vi "MapLocalToRemotePath.vi"(10 "appref":refnum<vi>, 11 "local path":path) -> (3 "remote path":path)   [LabVIEW 2020, in "NI_TargetHelper.lvlib" / "NetCPU.lvclass"]
uses:
  <vilib>/TargetSupport/NI_TargetHelper/NetCPU/NetCPU.lvclass
  <vilib>/Utility/sysdir.llb/System Directory Type.ctl
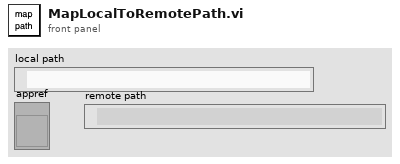
[diagram p1: front panel]
types:
  T1 = typedef "System Directory Type.ctl" = i32
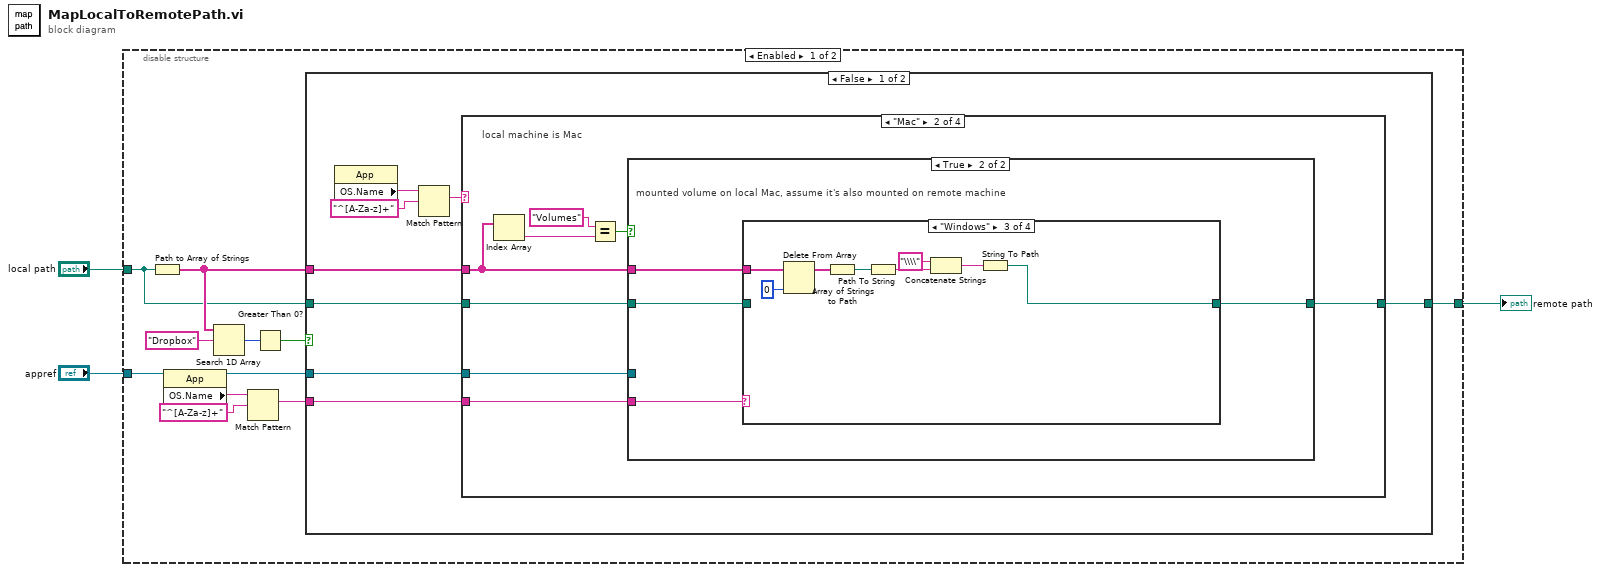
[diagram p0: block diagram]
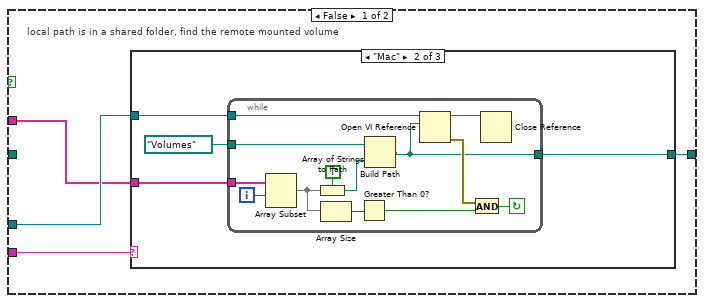
[diagram p3: hidden frame]
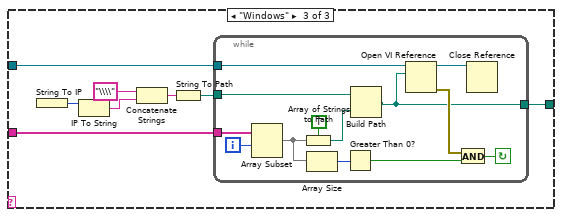
[diagram p5: hidden frame]
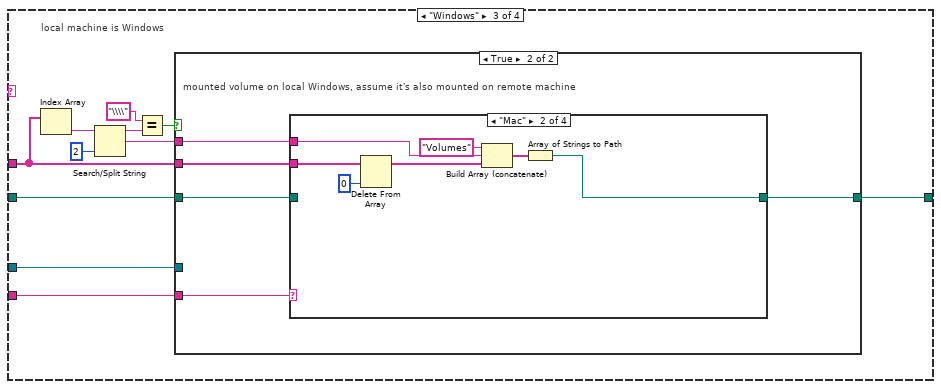
[diagram p9: hidden frame]
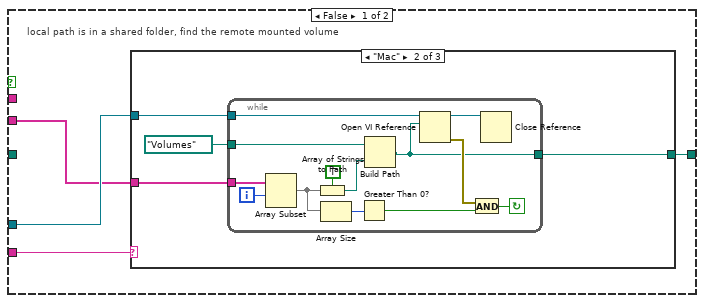
[diagram p10: hidden frame]
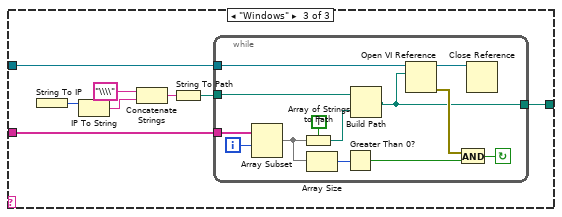
[diagram p12: hidden frame]
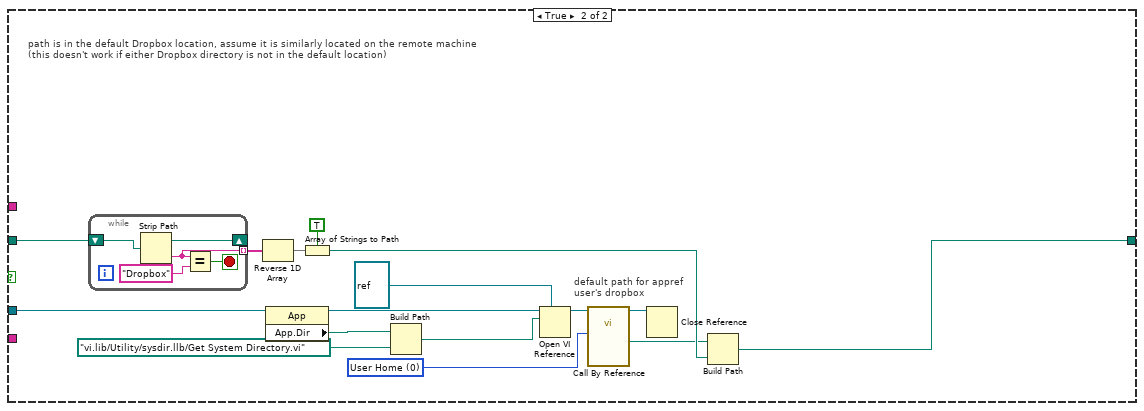
[diagram p17: hidden frame]
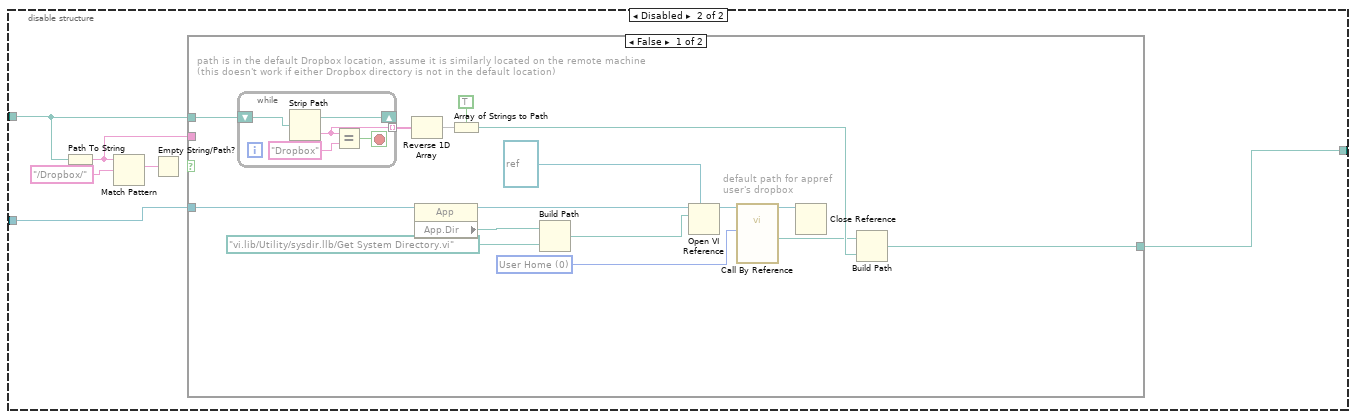
[diagram p18: hidden frame]
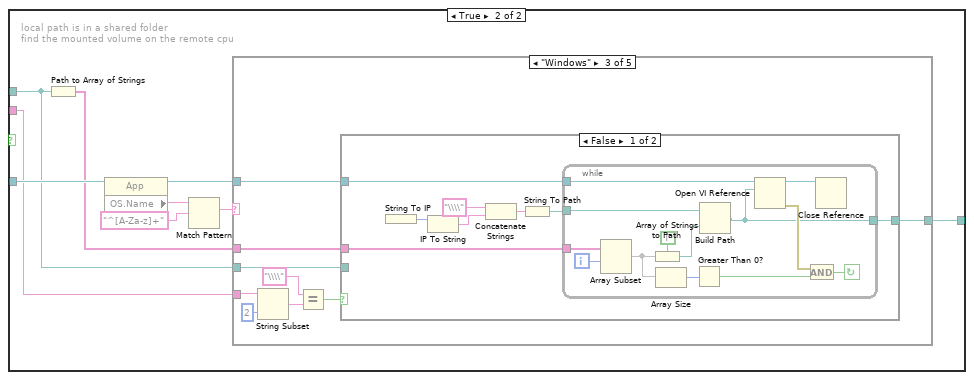
[diagram p19: hidden frame]
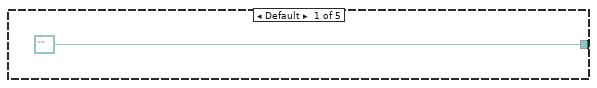
[diagram p20: hidden frame]
diagram:
  n1 = disable-structure shown="Enabled" {
    disable-tunnel: "appref" -> [w12 w174]
    disable-tunnel: "local path" -> [w4 w175]
    disable-tunnel: [w5 w173] -> w1
    frame Enabled {
      n2 = Path to Array of Strings(0:w4) -> (2:w7:string[])  [unwired: 1 out]
      n3 = property class="App"(reference=w12) -> (reference out=w10:refnum<vi>, "OS.Name"=w13:string)  [unwired: 1 in, 1 out]
      n4 = Search 1D Array(1D array=w7, element="Dropbox") -> (index of element=w9:i32)  [unwired: 1 in]
      n5 = Match Pattern(string=w13, regular expression="^[A-Za-z]+") -> (match substring=w11:string)  [unwired: 1 in, 3 out]
      n6 = Greater Than 0?(x=w9) -> (x > 0?=w6:bool)
      n7 = case shown="False" w6 {
        tunnel: w11 -> [w15 _]
        tunnel: w10 -> [w19 w153]
        tunnel: w4 -> [w18 w154]
        tunnel: w7 -> [w17 _]
        tunnel: [w16 w152] -> w5
        frame False {
          n8 = property class="App"() -> ("OS.Name"=w22:string)  [unwired: 2 in, 2 out]
          n9 = Match Pattern(string=w22, regular expression="^[A-Za-z]+") -> (match substring=w20:string)  [unwired: 1 in, 3 out]
          n10 = case shown="\"Mac\"" w20 {
            tunnel: w18 -> [_ w25 w92 _]
            tunnel: w15 -> [_ w27 w94 _]
            tunnel: [_ w26 w93 _] -> w16
            tunnel: w19 -> [_ w24 w91 _]
            tunnel: w17 -> [_ w23 w86 _]
            frame Default {
            }
            frame "Mac" {
              # "local machine is Mac"
              n11 = Index Array(array=w23) -> (element=w30:string)  [unwired: 1 in]
              n12 = Equal?(x="Volumes" ("y"), y=w30) -> (x = y?=w28:bool)
              n13 = case shown="True" w28 {
                tunnel: w27 -> [w32 w76]
                tunnel: [w31 w75] -> w26
                tunnel: w25 -> [_ w74]
                tunnel: w23 -> [w33 w73]
                tunnel: w24 -> [w34 _]
                frame False {
                  # "local path is in a shared folder, find the remote mounted volume"
                  n14 = case shown="\"Mac\"" w32 {
                    tunnel: w34 -> [_ w37 w53]
                    tunnel: w33 -> [_ w36 w52]
                    tunnel: [_ w35 w54] -> w31
                    frame Default {
                    }
                    frame "Mac" {
                      n15 = while {
                        tunnel: path "/Volumes" -> [w51]
                        tunnel: w37 -> [w50]
                        tunnel: w36 -> [w49]
                        tunnel: [w40] -> w35
                        i -> [w48]
                        stop <- w42 continue-if-true
                        n16 = Array Subset(array=w49, index=w48) -> (w46:string[])  [unwired: 1 in]
                        n17 = Array of Strings to Path(0:w46, 1:TRUE ("relative")) -> (2:w47:path)
                        n18 = Array Size(array=w46) -> (size(s)=w45:i32)
                        n19 = Greater Than 0?(x=w45) -> (x > 0?=w44:bool)
                        n20 = Build Path(base path=w51, name or relative path=w47) -> (appended path=w40:path)
                        n21 = Open VI Reference(application reference (local)=w50, vi path=w40) -> (vi reference=w39:refnum<vi>, error out=w43:errorcluster)  [unwired: 4 in]
                        n22 = And(x=w43, y=w44) -> (x .and. y?=w42:bool)
                        n23 = Close Reference(reference=w39) -> ()  [unwired: 1 in, 1 out]
                      }
                    }
                    frame "Windows" {
                      n24 = String To IP() -> (0:w59:u32)  [unwired: 1 in]
                      n25 = IP To String(2:w59) -> (0:w57:string)  [unwired: 1 in]
                      n26 = Concatenate Strings("\\\\" ("string"), w57) -> (w56:string)
                      n27 = String To Path(string=w56) -> (path=w55:path)
                      n28 = while {
                        tunnel: w55 -> [w72]
                        tunnel: w53 -> [w71]
                        tunnel: w52 -> [w70]
                        tunnel: [w61] -> w54
                        i -> [w69]
                        stop <- w63 continue-if-true
                        n29 = Array Subset(array=w70, index=w69) -> (w67:string[])  [unwired: 1 in]
                        n30 = Array of Strings to Path(0:w67, 1:TRUE ("relative")) -> (2:w68:path)
                        n31 = Array Size(array=w67) -> (size(s)=w66:i32)
                        n32 = Greater Than 0?(x=w66) -> (x > 0?=w65:bool)
                        n33 = Build Path(base path=w72, name or relative path=w68) -> (appended path=w61:path)
                        n34 = Open VI Reference(application reference (local)=w71, vi path=w61) -> (vi reference=w60:refnum<vi>, error out=w64:errorcluster)  [unwired: 4 in]
                        n35 = And(x=w64, y=w65) -> (x .and. y?=w63:bool)
                        n36 = Close Reference(reference=w60) -> ()  [unwired: 1 in, 1 out]
                      }
                    }
                  }
                }
                frame True {
                  # "mounted volume on local Mac, assume it's also mounted on remote machine"
                  n37 = case shown="\"Windows\"" w76 {
                    tunnel: [_ w77 w79 _] -> w75
                    tunnel: w74 -> [_ w77 _ _]
                    tunnel: w73 -> [_ _ w85 _]
                    frame Default {
                    }
                    frame "Mac" {
                    }
                    frame "Windows" {
                      n38 = Delete From Array(array=w85, index=0) -> (array with subset deleted=w84:string[])  [unwired: 1 in, 1 out]
                      n39 = Array of Strings to Path(0:w84) -> (2:w83:path)  [unwired: 1 in]
                      n40 = Path To String(path=w83) -> (string=w82:string)
                      n41 = Concatenate Strings("\\\\" ("string"), w82) -> (w80:string)
                      n42 = String To Path(string=w80) -> (path=w79:path)
                    }
                    frame "Linux" {
                    }
                  }
                }
              }
            }
            frame "Windows" {
              # "local machine is Windows"
              n43 = Index Array(array=w86) -> (element=w89:string)  [unwired: 1 in]
              n44 = Search/Split String(string=w89, offset (0)=2 ("length (rest)")) -> (substring before match=w88:string, match + rest of string=w87:string)  [unwired: 1 in, 1 out]
              n45 = Equal?(x="\\\\" ("y"), y=w88) -> (x = y?=w95:bool)
              n46 = case shown="True" w95 {
                tunnel: w94 -> [w98 w143]
                tunnel: [w97 w142] -> w93
                tunnel: w92 -> [_ w141]
                tunnel: w86 -> [w99 w140]
                tunnel: w91 -> [w100 _]
                tunnel: w87 -> [_ w139]
                frame False {
                  # "local path is in a shared folder, find the remote mounted volume"
                  n47 = case shown="\"Mac\"" w98 {
                    tunnel: w100 -> [_ w103 w119]
                    tunnel: w99 -> [_ w102 w118]
                    tunnel: [_ w101 w120] -> w97
                    frame Default {
                    }
                    frame "Mac" {
                      n48 = while {
                        tunnel: path "/Volumes" -> [w117]
                        tunnel: w103 -> [w116]
                        tunnel: w102 -> [w115]
                        tunnel: [w106] -> w101
                        i -> [w114]
                        stop <- w108 continue-if-true
                        n49 = Array Subset(array=w115, index=w114) -> (w112:string[])  [unwired: 1 in]
                        n50 = Array of Strings to Path(0:w112, 1:TRUE ("relative")) -> (2:w113:path)
                        n51 = Array Size(array=w112) -> (size(s)=w111:i32)
                        n52 = Greater Than 0?(x=w111) -> (x > 0?=w110:bool)
                        n53 = Build Path(base path=w117, name or relative path=w113) -> (appended path=w106:path)
                        n54 = Open VI Reference(application reference (local)=w116, vi path=w106) -> (vi reference=w105:refnum<vi>, error out=w109:errorcluster)  [unwired: 4 in]
                        n55 = And(x=w109, y=w110) -> (x .and. y?=w108:bool)
                        n56 = Close Reference(reference=w105) -> ()  [unwired: 1 in, 1 out]
                      }
                    }
                    frame "Windows" {
                      n57 = String To IP() -> (0:w125:u32)  [unwired: 1 in]
                      n58 = IP To String(2:w125) -> (0:w123:string)  [unwired: 1 in]
                      n59 = Concatenate Strings("\\\\" ("string"), w123) -> (w122:string)
                      n60 = String To Path(string=w122) -> (path=w121:path)
                      n61 = while {
                        tunnel: w121 -> [w138]
                        tunnel: w119 -> [w137]
                        tunnel: w118 -> [w136]
                        tunnel: [w127] -> w120
                        i -> [w135]
                        stop <- w129 continue-if-true
                        n62 = Array Subset(array=w136, index=w135) -> (w133:string[])  [unwired: 1 in]
                        n63 = Array of Strings to Path(0:w133, 1:TRUE ("relative")) -> (2:w134:path)
                        n64 = Array Size(array=w133) -> (size(s)=w132:i32)
                        n65 = Greater Than 0?(x=w132) -> (x > 0?=w131:bool)
                        n66 = Build Path(base path=w138, name or relative path=w134) -> (appended path=w127:path)
                        n67 = Open VI Reference(application reference (local)=w137, vi path=w127) -> (vi reference=w126:refnum<vi>, error out=w130:errorcluster)  [unwired: 4 in]
                        n68 = And(x=w130, y=w131) -> (x .and. y?=w129:bool)
                        n69 = Close Reference(reference=w126) -> ()  [unwired: 1 in, 1 out]
                      }
                    }
                  }
                }
                frame True {
                  # "mounted volume on local Windows, assume it's also mounted on remote machine"
                  n70 = case shown="\"Mac\"" w143 {
                    tunnel: [_ w144 w151 _] -> w142
                    tunnel: w141 -> [_ _ w151 _]
                    tunnel: w140 -> [_ w150 _ _]
                    tunnel: w139 -> [_ w147 _ _]
                    frame Default {
                    }
                    frame "Mac" {
                      n71 = Delete From Array(array=w150, index=0) -> (array with subset deleted=w148:string[])  [unwired: 1 in, 1 out]
                      n72 = Build Array (concatenate)("Volumes" ("element"), w147, w148) -> (w145:string[])
                      n73 = Array of Strings to Path(0:w145) -> (2:w144:path)  [unwired: 1 in]
                    }
                    frame "Windows" {
                    }
                    frame "Linux" {
                    }
                  }
                }
              }
            }
            frame "Linux" {
            }
          }
        }
        frame True {
          w162 = T1 0 items=["User Home"=0, "User Desktop"=1, "User Documents"=2, "User Application Data"=3, "User Preferences"=4, "User Temporary"=5, "Public Documents"=6, "Public Application Data"=7, "Public Preferences"=8, "Public Cache"=13, "System Core Libraries"=9, "System Installed Libraries"=10, "Application Files"=11, "Boot Volume Root"=12] ("system directory type")
          # "path is in the default Dropbox location, assume it is similarly located on the remote machine\n(this doesn't work if either Dropbox directory is not in the default location)"
          # "default path for appref \nuser's dropbox"
          n74 = while {
            shift-right: [w172] -> _
            shift-left: w154 -> [w169]
            tunnel: [w168] -> w161 mode=indexing
            stop <- w170 stop-if-true
            n75 = Strip Path(path=w169) -> (stripped path=w172:path, name=w168:string)
            n76 = Equal?(x=w168, y="Dropbox") -> (x = y?=w170:bool)
          }
          n77 = Reverse 1D Array(array=w161) -> (reversed array=w167:string[])
          n78 = property class="App"(reference=w153) -> (reference out=w159:refnum<vi>, "App.Dir"=w158:path)  [unwired: 1 in, 1 out]
          n79 = Array of Strings to Path(0:w167, 1:TRUE ("relative")) -> (2:w166:path)
          n80 = Build Path(base path=w158, name or relative path=path "vi.lib/Utility/sysdir.llb/Get System Directory.vi" ("vi path")) -> (appended path=w156:path)
          n81 = Open VI Reference(type specifier VI Refnum (for type only)=refnum<vi> refnum, application reference (local)=w159, vi path=w156) -> (vi reference=w164:refnum<vi>)  [unwired: 3 in, 1 out]
          n82 = call-by-ref "?"(reference=w164, "system directory type"=w162) -> (reference out=w163:refnum<vi>, "system directory"=w160:path)  [unwired: 11 in, 1 out]
          n83 = Close Reference(reference=w163) -> ()  [unwired: 1 in, 1 out]
          n84 = Build Path(base path=w160, name or relative path=w166) -> (appended path=w152:path)
        }
      }
    }
    frame Disabled {
      n85 = Path To String(path=w175) -> (string=w178:string)
      n86 = Match Pattern(string=w178, regular expression="/Dropbox/") -> (match substring=w177:string)  [unwired: 1 in, 3 out]
      n87 = Empty String/Path?(string/path=w177) -> ()  [unwired: 1 out]
      n88 = case shown="False" {
        selector: _ -> [_ _]
        tunnel: w175 -> [w193 w201]
        tunnel: [w194 w204] -> w173
        tunnel: w174 -> [w183 w205]
        tunnel: w178 -> [_ w200]
        frame False {
          w187 = T1 0 items=["User Home"=0, "User Desktop"=1, "User Documents"=2, "User Application Data"=3, "User Preferences"=4, "User Temporary"=5, "Public Documents"=6, "Public Application Data"=7, "Public Preferences"=8, "Public Cache"=13, "System Core Libraries"=9, "System Installed Libraries"=10, "Application Files"=11, "Boot Volume Root"=12] ("system directory type")
          # "path is in the default Dropbox location, assume it is similarly located on the remote machine\n(this doesn't work if either Dropbox directory is not in the default location)"
          # "default path for appref \nuser's dropbox"
          n89 = while {
            shift-right: [w199] -> _
            shift-left: w193 -> [w196]
            tunnel: [w195] -> w186 mode=indexing
            stop <- w197 stop-if-true
            n90 = Strip Path(path=w196) -> (stripped path=w199:path, name=w195:string)
            n91 = Equal?(x=w195, y="Dropbox") -> (x = y?=w197:bool)
          }
          n92 = Reverse 1D Array(array=w186) -> (reversed array=w192:string[])
          n93 = property class="App"(reference=w183) -> (reference out=w184:refnum<vi>, "App.Dir"=w182:path)  [unwired: 1 in, 1 out]
          n94 = Array of Strings to Path(0:w192, 1:TRUE ("relative")) -> (2:w191:path)
          n95 = Build Path(base path=w182, name or relative path=path "vi.lib/Utility/sysdir.llb/Get System Directory.vi" ("vi path")) -> (appended path=w180:path)
          n96 = Open VI Reference(type specifier VI Refnum (for type only)=refnum<vi> refnum, application reference (local)=w184, vi path=w180) -> (vi reference=w189:refnum<vi>)  [unwired: 3 in, 1 out]
          n97 = call-by-ref "?"(reference=w189, "system directory type"=w187) -> (reference out=w188:refnum<vi>, "system directory"=w185:path)  [unwired: 11 in, 1 out]
          n98 = Close Reference(reference=w188) -> ()  [unwired: 1 in, 1 out]
          n99 = Build Path(base path=w185, name or relative path=w191) -> (appended path=w194:path)
        }
        frame True {
          # "local path is in a shared folder\nfind the mounted volume on the remote cpu"
          n100 = Path to Array of Strings(0:w201) -> (2:w202:string[])  [unwired: 1 out]
          n101 = property class="App"(reference=w205) -> (reference out=w203:refnum<vi>, "OS.Name"=w208:string)  [unwired: 1 in, 1 out]
          n102 = Match Pattern(string=w208, regular expression="^[A-Za-z]+") -> (match substring=w206:string)  [unwired: 1 in, 3 out]
          n103 = case shown="\"Windows\"" w206 {
            tunnel: [path "" w216 w243 w268 w289] -> w204
            tunnel: w203 -> [_ w215 w242 w266 w291]
            tunnel: w202 -> [_ w214 w241 w269 w290]
            tunnel: w201 -> [_ w210 w235 _ _]
            tunnel: w200 -> [_ _ w240 _ _]
            frame Default {
            }
            frame "Mac" {
              n104 = Index Array(array=w214) -> (element=w213:string)  [unwired: 1 in]
              n105 = Equal?(x="Volumes" ("y"), y=w213) -> (x = y?=w211:bool)
              n106 = case shown="False" w211 {
                tunnel: [w219 w234] -> w216
                tunnel: w215 -> [w218 _]
                tunnel: w214 -> [w217 _]
                tunnel: w210 -> [_ w234]
                frame False {
                  n107 = while {
                    tunnel: path "/Volumes" -> [w233]
                    tunnel: w218 -> [w232]
                    tunnel: w217 -> [w231]
                    tunnel: [w222] -> w219
                    i -> [w230]
                    stop <- w224 continue-if-true
                    n108 = Array Subset(array=w231, index=w230) -> (w228:string[])  [unwired: 1 in]
                    n109 = Array of Strings to Path(0:w228, 1:TRUE ("relative")) -> (2:w229:path)
                    n110 = Array Size(array=w228) -> (size(s)=w227:i32)
                    n111 = Greater Than 0?(x=w227) -> (x > 0?=w226:bool)
                    n112 = Build Path(base path=w233, name or relative path=w229) -> (appended path=w222:path)
                    n113 = Open VI Reference(application reference (local)=w232, vi path=w222) -> (vi reference=w221:refnum<vi>, error out=w225:errorcluster)  [unwired: 4 in]
                    n114 = And(x=w225, y=w226) -> (x .and. y?=w224:bool)
                    n115 = Close Reference(reference=w221) -> ()  [unwired: 1 in, 1 out]
                  }
                }
                frame True {
                }
              }
            }
            frame "Windows" {
              n116 = String Subset(string=w240, length (rest)=2 ("length (rest)")) -> (substring=w238:string)  [unwired: 1 in]
              n117 = Equal?(x="\\\\", y=w238) -> (x = y?=w236:bool)
              n118 = case shown="False" w236 {
                tunnel: [w251 w265] -> w243
                tunnel: w242 -> [w250 _]
                tunnel: w241 -> [w249 _]
                tunnel: w235 -> [_ w265]
                frame False {
                  n119 = String To IP() -> (0:w248:u32)  [unwired: 1 in]
                  n120 = IP To String(2:w248) -> (0:w246:string)  [unwired: 1 in]
                  n121 = Concatenate Strings("\\\\" ("string"), w246) -> (w245:string)
                  n122 = String To Path(string=w245) -> (path=w244:path)
                  n123 = while {
                    tunnel: w244 -> [w264]
                    tunnel: w250 -> [w263]
                    tunnel: w249 -> [w262]
                    tunnel: [w253] -> w251
                    i -> [w261]
                    stop <- w255 continue-if-true
                    n124 = Array Subset(array=w262, index=w261) -> (w259:string[])  [unwired: 1 in]
                    n125 = Array of Strings to Path(0:w259, 1:TRUE ("relative")) -> (2:w260:path)
                    n126 = Array Size(array=w259) -> (size(s)=w258:i32)
                    n127 = Greater Than 0?(x=w258) -> (x > 0?=w257:bool)
                    n128 = Build Path(base path=w264, name or relative path=w260) -> (appended path=w253:path)
                    n129 = Open VI Reference(application reference (local)=w263, vi path=w253) -> (vi reference=w252:refnum<vi>, error out=w256:errorcluster)  [unwired: 4 in]
                    n130 = And(x=w256, y=w257) -> (x .and. y?=w255:bool)
                    n131 = Close Reference(reference=w252) -> ()  [unwired: 1 in, 1 out]
                  }
                }
                frame True {
                  # "Assume if the path starts with \\\\ we're in a shared location\nthat's accessible to all machines."
                }
              }
            }
            frame "Windowsold" {
              n132 = String To IP() -> (0:w272:u32)  [unwired: 1 in]
              n133 = IP To String(2:w272) -> (0:w270:string)  [unwired: 1 in]
              n134 = Concatenate Strings("\\\\" ("string"), w270) -> (w267:string)
              n135 = while {
                tunnel: w267 -> [w276]
                tunnel: w266 -> [w284]
                tunnel: w269 -> [w283]
                tunnel: [w274] -> w268
                i -> [w282]
                stop <- w278 continue-if-true
                n136 = Array Subset(array=w283, index=w282) -> (w277:string[])  [unwired: 1 in]
                n137 = for {
                  tunnel: w277 -> [w286] mode=indexing
                  shift-right: [w288] -> w275
                  shift-left: w276 -> [w287]
                  n138 = Concatenate Strings(w287, "\\" ("string"), w286) -> (w288:string)
                }
                n139 = Array Size(array=w277) -> (size(s)=w281:i32)
                n140 = Greater Than 0?(x=w281) -> (x > 0?=w280:bool)
                n141 = String To Path(string=w275) -> (path=w274:path)
                n142 = Open VI Reference(application reference (local)=w284, vi path=w274) -> (vi reference=w273:refnum<vi>, error out=w279:errorcluster)  [unwired: 4 in]
                n143 = And(x=w279, y=w280) -> (x .and. y?=w278:bool)
                n144 = Close Reference(reference=w273) -> ()  [unwired: 1 in, 1 out]
              }
            }
            frame "Linux" {
              n145 = while {
                tunnel: path "" -> [w305]
                tunnel: w291 -> [w304]
                tunnel: w290 -> [w303]
                tunnel: [w294] -> w289
                i -> [w302]
                stop <- w296 continue-if-true
                n146 = Array Subset(array=w303, index=w302) -> (w300:string[])  [unwired: 1 in]
                n147 = Array of Strings to Path(0:w300, 1:TRUE ("relative")) -> (2:w301:path)
                n148 = Array Size(array=w300) -> (size(s)=w299:i32)
                n149 = Greater Than 0?(x=w299) -> (x > 0?=w298:bool)
                n150 = Build Path(base path=w305, name or relative path=w301) -> (appended path=w294:path)
                n151 = Open VI Reference(application reference (local)=w304, vi path=w294) -> (vi reference=w293:refnum<vi>, error out=w297:errorcluster)  [unwired: 4 in]
                n152 = And(x=w297, y=w298) -> (x .and. y?=w296:bool)
                n153 = Close Reference(reference=w293) -> ()  [unwired: 1 in, 1 out]
              }
            }
          }
        }
      }
    }
  }
  "remote path" <- w1
